vi "Find Octave Executable Older Versions.vi"() -> (1 "Found executable?":bool, 3 "Executable path":path)   [LabVIEW 2020, in "GOLPI library.lvlib"]
doc: "Returns valid path with GNU Octave executable based on known default installation paths for versions 3,4,5 and 6."
uses:
  GOLPI library.lvlib
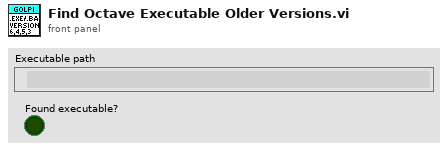
[diagram p1: front panel]
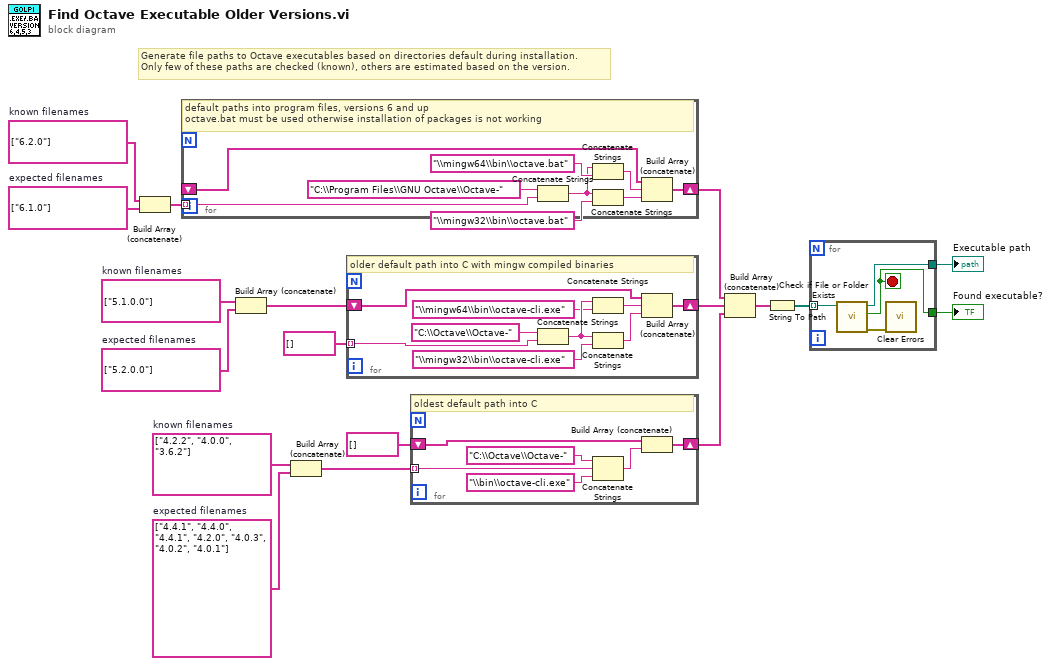
[diagram p0: block diagram]
diagram:
  w13 = string[] ["6.1.0"]  # expected filenames
  w8 = string[] ["5.2.0.0"]  # expected filenames
  w5 = string[] ["4.4.1", "4.4.0", "4.4.1", "4.2.0", "4.0.3", "4.0.2", "4.0.1"]  # expected filenames
  w9 = string[] ["5.1.0.0"]  # known filenames
  w12 = string[] ["6.2.0"]  # known filenames
  w4 = string[] ["4.2.2", "4.0.0", "3.6.2"]  # known filenames
  # "Generate file paths to Octave executables based on directories default during installation.\nOnly few of these paths are checked (known), others are estimated based on the version."
  n1 = Build Array (concatenate)(w12, w13) -> (w14:string[])
  n2 = for {
    tunnel: w14 -> [w25] mode=indexing
    shift-right: [w26] -> w15
    shift-left: _ -> [w27]
    # "default paths into program files, versions 6 and up\noctave.bat must be used otherwise installation of packages is not working"
    n3 = Concatenate Strings("C:\\Program Files\\GNU Octave\\Octave-" ("format string"), w25) -> (w22:string)
    n4 = Concatenate Strings(w22, "\\mingw64\\bin\\octave.bat" ("format string")) -> (w20:string)
    n5 = Concatenate Strings(w22, "\\mingw32\\bin\\octave.bat" ("format string")) -> (w19:string)
    n6 = Build Array (concatenate)(w27, w20, w19) -> (w26:string[])
  }
  n7 = Build Array (concatenate)(w9, w8) -> (w10:string[])
  n8 = Build Array (concatenate)(w4, w5) -> (w6:string[])
  n9 = for {
    tunnel: string[] [] ("appended array") -> [w34] mode=indexing
    shift-right: [w35] -> w16
    shift-left: w10 -> [w36]
    # "older default path into C with mingw compiled binaries"
    n10 = Concatenate Strings("C:\\Octave\\Octave-" ("format string"), w34) -> (w32:string)
    n11 = Concatenate Strings(w32, "\\mingw64\\bin\\octave-cli.exe" ("format string")) -> (w29:string)
    n12 = Concatenate Strings(w32, "\\mingw32\\bin\\octave-cli.exe" ("format string")) -> (w28:string)
    n13 = Build Array (concatenate)(w36, w29, w28) -> (w35:string[])
  }
  n14 = for {
    tunnel: w6 -> [w39] mode=indexing
    shift-right: [w41] -> w17
    shift-left: string[] [] ("appended array") -> [w42]
    # "oldest default path into C"
    n15 = Concatenate Strings("C:\\Octave\\Octave-" ("format string"), w39, "\\bin\\octave-cli.exe" ("format string")) -> (w40:string)
    n16 = Build Array (concatenate)(w42, w40) -> (w41:string[])
  }
  n17 = Build Array (concatenate)(w15, w16, w17) -> (w18:string[])
  n18 = String To Path(string=w18) -> (path=w3:path[])
  n19 = for {
    tunnel: w3 -> [w46] mode=indexing
    tunnel: [w44] -> w2
    tunnel: [w43] -> w1
    stop <- w43 stop-if-true
    n20 = call <vilib>:"Check if File or Folder Exists.vi"("path"=w46) -> ("error out"=w45:errorcluster, "file or folder exists?"=w43:bool, "dup path"=w44:path)  [unwired: 8 in]
    n21 = call <vilib>:"Clear Errors.vi"("error in (no error)"=w45) -> ()  [unwired: 5 in, 2 out]
  }
  "Executable path" <- w2
  "Found executable?" <- w1
